vi "Using Analysis tools (Waveform data type).vi"() -> ()   [LabVIEW 2019]
uses:
  <vilib>/DAQmx/read.llb/DAQmx Read (Analog Wfm 1Chan NSamp).vi
  <vilib>/DAQmx/create/channels.llb/DAQmx Create Channel (AI-Temperature-Thermocouple).vi
  <vilib>/DAQmx/configure/timing.llb/DAQmx Timing (Sample Clock).vi
  <vilib>/DAQmx/miscellaneous.llb/DAQmx Fill In Error Info.vi
  <vilib>/measure/mascope.llb/Amplitude and Levels N chan.vi
  <resource>/objmgr/daqmx.rc
  <vilib>/measure/NI_MAPro.lvlib
panel:
  out "min value":dbl
  out "max value":dbl
  out "Acquired Signal":waveform(dbl)(graph)
  in  "Stop":bool
  out "Actual Sample Rate (Hz)":dbl
  in  "Number of Samples":i32=1000
  in  "Desired Sample Rate (Hz)":dbl=1000.0
  in  "Physical Channel":tag="PCI-6221/ai0"
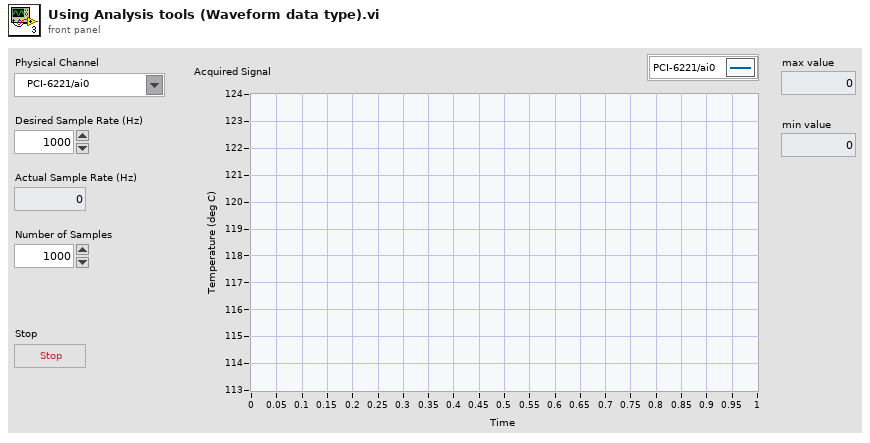
[diagram p1: front panel]
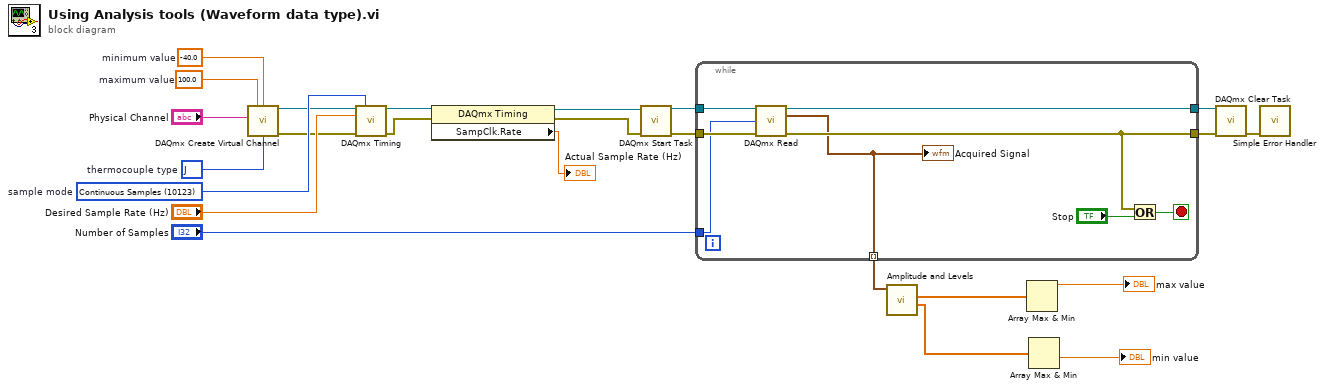
[diagram p0: block diagram]
diagram:
  w1 = 10072 items=["J"=10072, "K"=10073, "N"=10077, "R"=10082, "S"=10085, "T"=10086, "B"=10047, "E"=10055]  # thermocouple type
  w21 = 10123 items=["Finite Samples"=10178, "Continuous Samples"=10123, "Hardware Timed Single Point"=12522]  # sample mode
  w23 = 100.0  # maximum value
  w24 = -40.0  # minimum value
  n1 = call-poly <vilib>:"DAQmx Create Virtual Channel.vi"("maximum value"=w23, "minimum value"=w24, "physical channels"="Physical Channel", "thermocouple type"=w1) -> ("task out"=w19:refnum<k21>, "error out"=w18:errorcluster)  [unwired: 10 in]
  n2 = call-poly <vilib>:"DAQmx Timing.vi"("task/channels in"=w19, "sample mode"=w21, "rate"="Desired Sample Rate (Hz)", "error in"=w18) -> ("task out"=w17:refnum<k21>, "error out"=w16:errorcluster)  [unwired: 10 in]
  n3 = property class="DAQmx Timing"(reference=w17, error in=w16) -> (reference out=w14:refnum<k21>, error out=w13:errorcluster, "SampClk.Rate"=→"Actual Sample Rate (Hz)":dbl)
  n4 = call <vilib>:"DAQmx Start Task.vi"("task/channels in"=w14, "error in"=w13) -> ("task out"=w12:refnum<k21>, "error out"=w11:errorcluster)  [unwired: 12 in]
  n5 = while {
    tunnel: w12 -> [w32]
    tunnel: w11 -> [w31]
    tunnel: "Number of Samples" -> [w30]
    tunnel: [w29] -> w9
    tunnel: [w28] -> w8
    tunnel: [w25] -> w6 mode=indexing
    stop <- w26 stop-if-true
    n6 = call-poly <vilib>:"DAQmx Read.vi"("task/channels in"=w32, "number of samples per channel"=w30, "error in"=w31) -> ("task out"=w29:refnum<k21>, "data"=w25:waveform(dbl), "error out"=w28:errorcluster)  [unwired: 10 in]
    "Acquired Signal" <- w25
    n7 = Or(x=w28, y="Stop") -> (x .or. y?=w26:bool)
  }
  n8 = call-poly <vilib>:"Amplitude and Levels.vi"("signal(s) in"=w6) -> ("low state level"=w2:dbl[], "high state level"=w3:dbl[])  [unwired: 7 in, 2 out]
  n9 = Array Max & Min(array=w3) -> (max value=→"max value":dbl)  [unwired: 3 out]
  n10 = Array Max & Min(array=w2) -> (min value=→"min value":dbl)  [unwired: 3 out]
  n11 = call <vilib>:"DAQmx Clear Task.vi"("task in"=w9, "error in"=w8) -> ("error out"=w7:errorcluster)  [unwired: 13 in]
  n12 = call <vilib>:"Simple Error Handler.vi"("error in (no error)"=w7) -> ()  [unwired: 4 in, 5 out]
